vi "Execute.vi"(10 "Test Runner V2 in":refnum<class "Runnable.lvclass">) -> ()   [LabVIEW 2020, in "Parallell Test Runner.lvclass"]
uses:
  Parallell Test Runner.lvclass
  Run/Runnable.lvclass
  Parallell Test Runner.lvclass/Parallell Test Runner.ctl
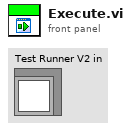
[diagram p1: front panel]
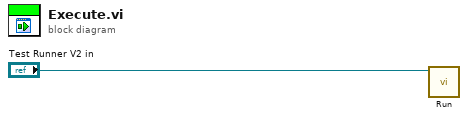
[diagram p0: block diagram]
diagram:
  n1 = call-dynamic "Run.vi"("Run in"="Test Runner V2 in") -> ()  [unwired: 9 in, 2 out]
